vi "Basic.vi"() -> ()   [LabVIEW 2020]
uses:
  Typedef Employee.ctl
panel:
  in  "employee 25":T1={"Name"="Atul Ghumade", "Age"=29, "Salary"=100000, "Gender"=TRUE, "Hobby"="Atul Ghumade"}
  in  "employee 24":T1={"Name"="Atul Ghumade", "Age"=29, "Salary"=100000, "Gender"=TRUE, "Hobby"="Atul Ghumade"}
  in  "employee 23":T1={"Name"="Atul Ghumade", "Age"=29, "Salary"=100000, "Gender"=TRUE, "Hobby"="Atul Ghumade"}
  in  "employee 22":T1={"Name"="Atul Ghumade", "Age"=29, "Salary"=100000, "Gender"=TRUE, "Hobby"="Atul Ghumade"}
  in  "employee 21":T1={"Name"="Atul Ghumade", "Age"=29, "Salary"=100000, "Gender"=TRUE, "Hobby"="Atul Ghumade"}
  in  "employee 20":T1={"Name"="Atul Ghumade", "Age"=29, "Salary"=100000, "Gender"=TRUE, "Hobby"="Atul Ghumade"}
  in  "employee 19":T1={"Name"="Atul Ghumade", "Age"=29, "Salary"=100000, "Gender"=TRUE, "Hobby"="Atul Ghumade"}
  in  "employee 18":T1={"Name"="Atul Ghumade", "Age"=29, "Salary"=100000, "Gender"=TRUE, "Hobby"="Atul Ghumade"}
  in  "employee 17":T1={"Name"="Atul Ghumade", "Age"=29, "Salary"=100000, "Gender"=TRUE, "Hobby"="Atul Ghumade"}
  in  "employee 16":T1={"Name"="Atul Ghumade", "Age"=29, "Salary"=100000, "Gender"=TRUE, "Hobby"="Atul Ghumade"}
  in  "employee 15":T1={"Name"="Atul Ghumade", "Age"=29, "Salary"=100000, "Gender"=TRUE, "Hobby"="Atul Ghumade"}
  in  "employee 14":T1={"Name"="Atul Ghumade", "Age"=29, "Salary"=100000, "Gender"=TRUE, "Hobby"="Atul Ghumade"}
  in  "employee 13":T1={"Name"="Atul Ghumade", "Age"=29, "Salary"=100000, "Gender"=TRUE, "Hobby"="Atul Ghumade"}
  in  "employee 12":T1={"Name"="Atul Ghumade", "Age"=29, "Salary"=100000, "Gender"=TRUE, "Hobby"="Atul Ghumade"}
  in  "employee 11":T1={"Name"="Atul Ghumade", "Age"=29, "Salary"=100000, "Gender"=TRUE, "Hobby"="Atul Ghumade"}
  in  "employee 10":T1={"Name"="Atul Ghumade", "Age"=29, "Salary"=100000, "Gender"=TRUE, "Hobby"="Atul Ghumade"}
  in  "employee 9":T1={"Name"="Atul Ghumade", "Age"=29, "Salary"=100000, "Gender"=TRUE, "Hobby"="Atul Ghumade"}
  in  "employee 8":T1={"Name"="Atul Ghumade", "Age"=29, "Salary"=100000, "Gender"=TRUE, "Hobby"="Atul Ghumade"}
  in  "employee 7":T1={"Name"="Atul Ghumade", "Age"=29, "Salary"=100000, "Gender"=TRUE, "Hobby"="Atul Ghumade"}
  in  "employee 6":T1={"Name"="Atul Ghumade", "Age"=29, "Salary"=100000, "Gender"=TRUE, "Hobby"="Atul Ghumade"}
  in  "employee 5":T1={"Name"="Atul Ghumade", "Age"=29, "Salary"=100000, "Gender"=TRUE, "Hobby"="Atul Ghumade"}
  in  "employee 4":T1={"Name"="Atul Ghumade", "Age"=29, "Salary"=100000, "Gender"=TRUE, "Hobby"="Atul Ghumade"}
  in  "employee 3":T1={"Name"="Atul Ghumade", "Age"=29, "Salary"=100000, "Gender"=TRUE, "Hobby"="Atul Ghumade"}
  in  "employee 2":T1={"Name"="Atul Ghumade", "Age"=29, "Salary"=100000, "Gender"=TRUE, "Hobby"="Atul Ghumade"}
  in  "employee":T1={"Name"="Atul Ghumade", "Age"=29, "Salary"=100000, "Gender"=TRUE, "Hobby"="Atul Ghumade"}
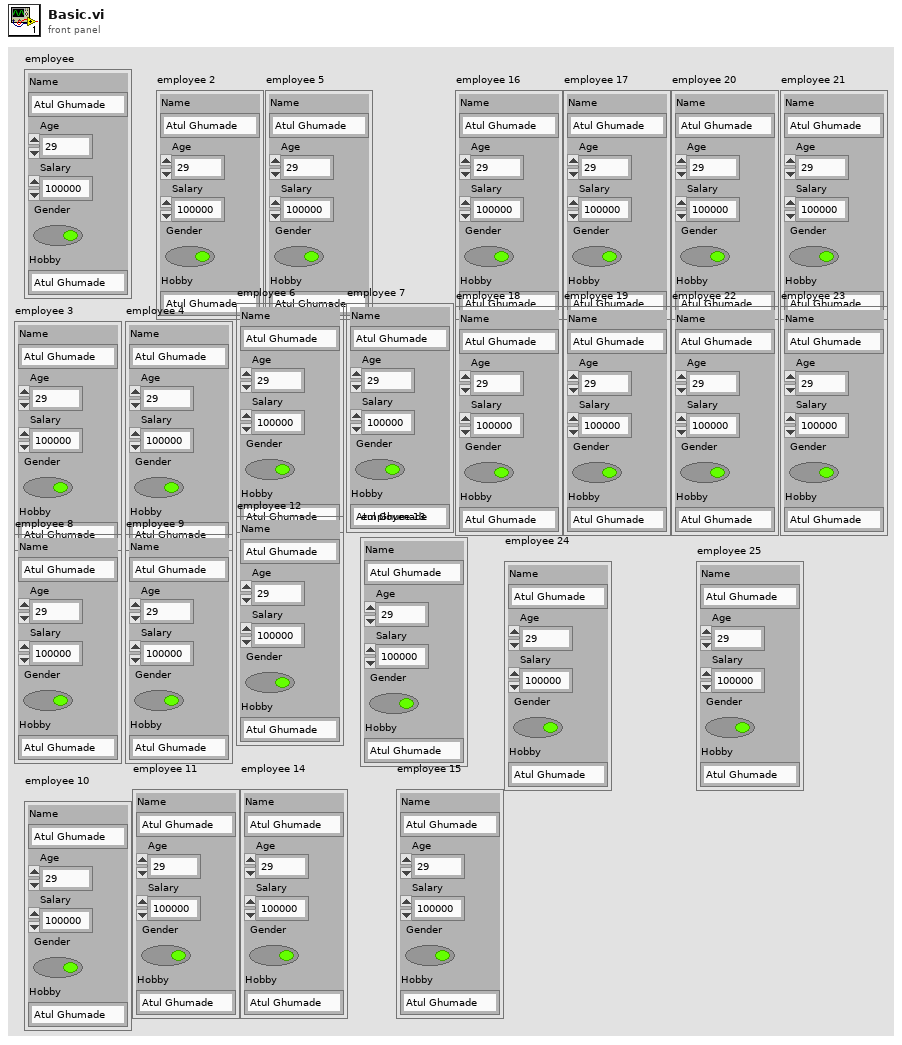
[diagram p1: front panel]
types:
  T1 = typedef "Typedef Employee.ctl" = cluster{"Name":string, "Age":u8, "Salary":u32, "Gender":bool, "Hobby":string}
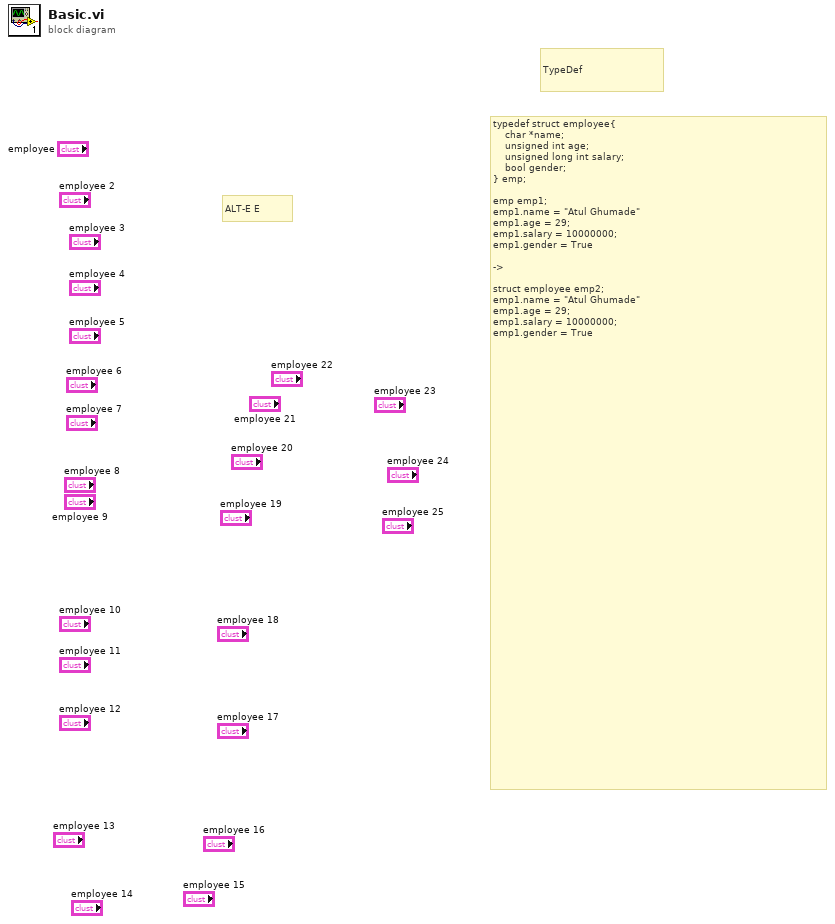
[diagram p0: block diagram]
diagram:
  # "ALT-E E"
  # "typedef struct employee{\n    char *name;\n    unsigned int age;\n    unsigned long int salary;\n    bool gender;\n} emp;\n\nemp emp1;\nemp1.name = \"Atul Ghumade\"\nemp1.age = 29;\nemp1.salary = 10000000;\nemp1.gender = True\n\n->\n\nstruct employee emp2;\nemp1.name = \"Atul Ghumade\"\nemp1.age = 29;\nemp1.salary = 10000000;\nemp1.gender = True"
  # "TypeDef"
